vi "串口调试程序.VI"() -> ()   [LabVIEW 2015]
uses:
  <vilib>/Instr/_visa.llb/VISA Configure Serial Port (Instr).vi
panel:
  out "当前时间":timestamp
  in  "清零":bool
  out "接收字节数":u32
  out "发送字节数":u32
  in  "Boolean 9":bool
  in  "毫秒倍数":u32=100 min=2 step=1
  in  "自动发送":bool
  in  "十六进制发送":bool
  in  "OK Button 2":bool
  in  "十六进制接收":bool
  in  "Boolean 8":bool
  in  "退出":bool
  out "接收数据区：":string
  in  "发送数据区：":string
  in  "发送":bool
  in  "打开":bool caption="stop"
  in  "校验位：":u16(ring) items=["  无校验", "  奇校验", "  偶校验"]
  in  "波特率：":u16(ring)=11 items=["   300", "   600", "   1200", "   2400", "   4800   ", "   9600", "   19200", "   38400", "   43000", "   56000", "   57600", "   115200"]
  in  "通讯口：":u16(ring) items=["   com1", "   com2", "   com3", "   com4", "   com5"]
  # "通讯口设置："
  # "接收数据设置："
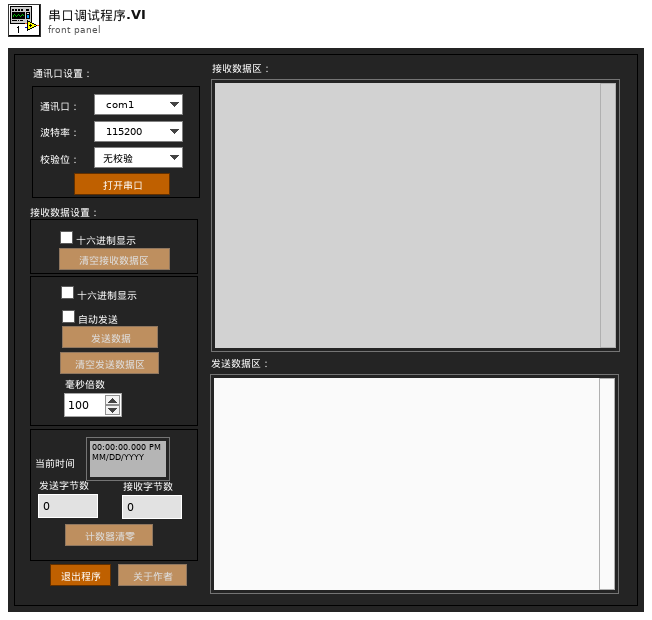
[diagram p1: front panel]
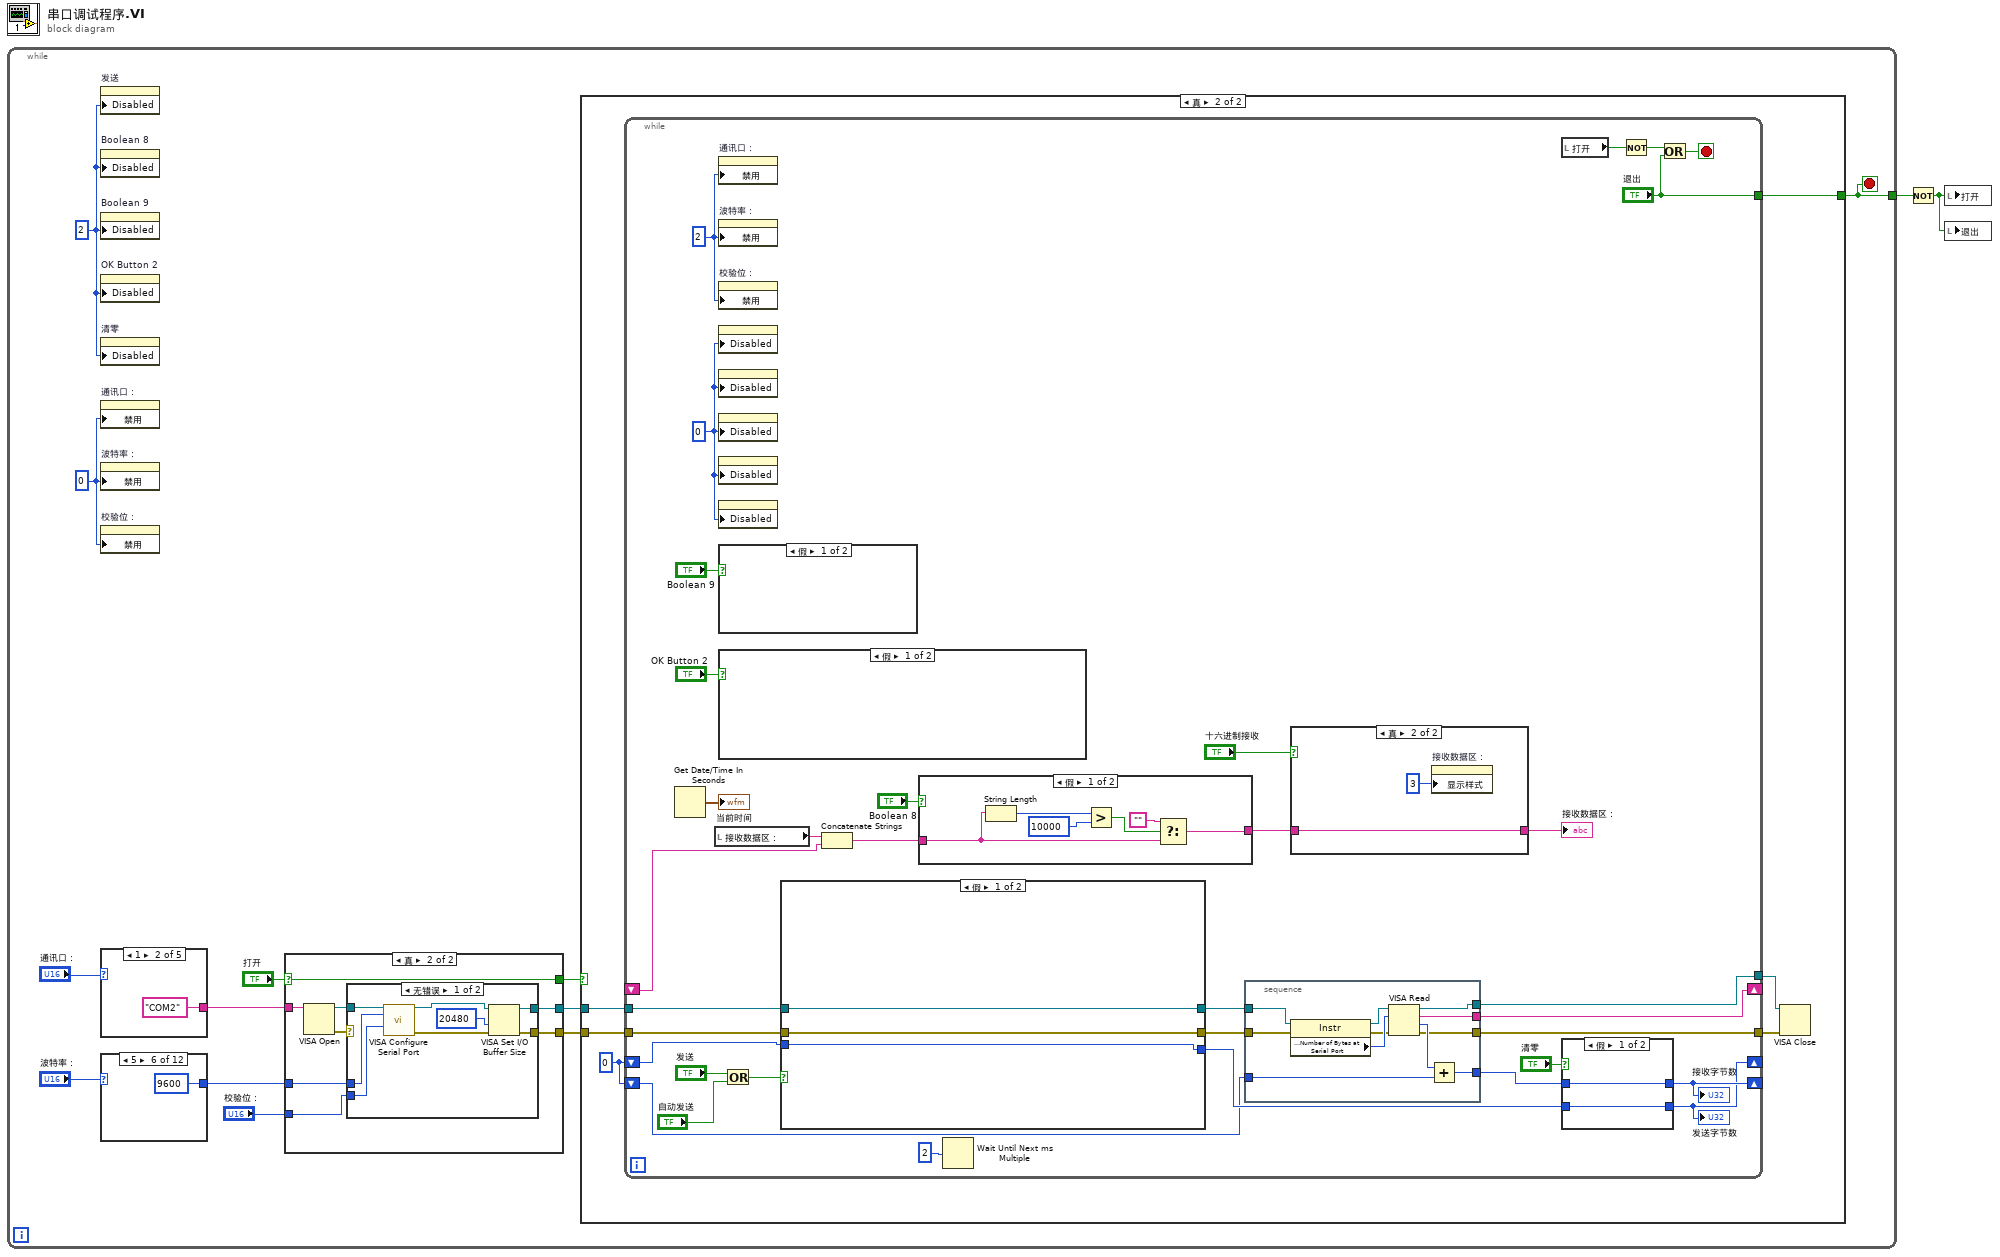
[diagram p0: block diagram]
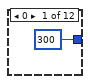
[diagram p2: hidden frame]
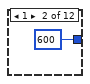
[diagram p3: hidden frame]
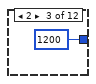
[diagram p4: hidden frame]
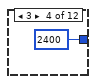
[diagram p5: hidden frame]
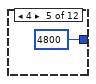
[diagram p6: hidden frame]
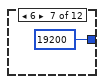
[diagram p7: hidden frame]
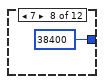
[diagram p8: hidden frame]
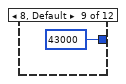
[diagram p9: hidden frame]
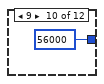
[diagram p10: hidden frame]
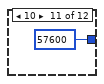
[diagram p11: hidden frame]
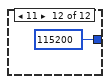
[diagram p12: hidden frame]
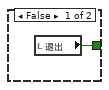
[diagram p13: hidden frame]
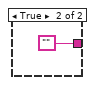
[diagram p14: hidden frame]
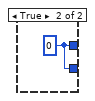
[diagram p15: hidden frame]
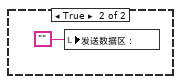
[diagram p16: hidden frame]
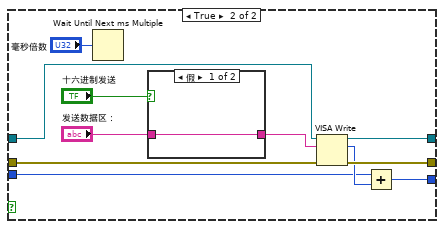
[diagram p17: hidden frame]
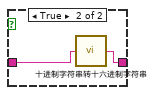
[diagram p18: hidden frame]
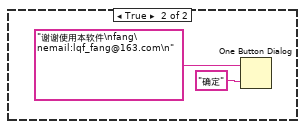
[diagram p19: hidden frame]
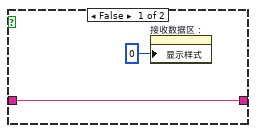
[diagram p20: hidden frame]
diagram:
  n1 = while {
    tunnel: [w7] -> w2
    stop <- w7 stop-if-true
    w5 = 2
    w9 = 0
    n2 = property on="发送" class="Bool"("Disabled"=w5) -> ()  [unwired: 2 in, 2 out]
    n3 = property on="Boolean 8" class="Bool"("Disabled"=w5) -> ()  [unwired: 2 in, 2 out]
    n4 = property on="Boolean 9" class="Bool"("Disabled"=w5) -> ()  [unwired: 2 in, 2 out]
    n5 = property on="OK Button 2" class="Bool"("Disabled"=w5) -> ()  [unwired: 2 in, 2 out]
    n6 = property on="清零" class="Bool"("Disabled"=w5) -> ()  [unwired: 2 in, 2 out]
    n7 = property on="通讯口：" class="Ring (严格)"("禁用"=w9) -> ()  [unwired: 2 in, 2 out]
    n8 = property on="波特率：" class="Ring (严格)"("禁用"=w9) -> ()  [unwired: 2 in, 2 out]
    n9 = property on="校验位：" class="Ring (严格)"("禁用"=w9) -> ()  [unwired: 2 in, 2 out]
    n10 = case shown="1" "通讯口：" {
      tunnel: ["COM1" "COM2" "COM3" "COM4" "COM5"] -> w8
      frame 0, Default {
      }
      frame 1 {
      }
      frame 2 {
      }
      frame 3 {
      }
      frame 4 {
      }
    }
    n11 = case shown="5" "波特率：" {
      tunnel: [300 600 1200 2400 4800 9600 19200 38400 43000 56000 57600 115200] -> w3
      frame 0 {
      }
      frame 1 {
      }
      frame 2 {
      }
      frame 3 {
      }
      frame 4 {
      }
      frame 5 {
      }
      frame 6 {
      }
      frame 7 {
      }
      frame 8, Default {
      }
      frame 9 {
      }
      frame 10 {
      }
      frame 11 {
      }
    }
    n12 = case shown="真" "打开" {
      selector: "打开" -> [w113 w121]
      tunnel: w3 -> [_ w117]
      tunnel: [w113 w121] -> w12
      tunnel: [_ w115] -> w11
      tunnel: [_ w114] -> w10
      tunnel: w8 -> [_ w120]
      tunnel: "校验位：" -> [_ w116]
      frame False {
      }
      frame True {
        n13 = VISA Open(VISA resource name=w120) -> (VISA resource name=w118:refnum<visa-resource-name>, error out=w119:errorcluster)  [unwired: 4 in]
        n14 = case shown="无错误" w119 {
          tunnel: w118 -> [w129 _]
          tunnel: w117 -> [w128 _]
          tunnel: w116 -> [w127 _]
          tunnel: [w123 _] -> w115
          tunnel: [w124 _] -> w114
          frame No Error {
            n15 = call-poly "VISA Configure Serial Port"("VISA resource name"=w129, "baud rate (9600)"=w128, "parity (0:none)"=w127) -> ("VISA resource name out"=w126:refnum<visa-resource-name>, "error out"=w125:errorcluster)  [unwired: 11 in]
            n16 = VISA Set I/O Buffer Size(VISA resource name=w126, size (4096)=u32 20480 ("大小(4096)"), error in (no error)=w125) -> (VISA resource name out=w123:refnum<visa-resource-name>, error out=w124:errorcluster)  [unwired: 1 in]
          }
          frame Error {
            n17 = One Button Dialog(message="ERROR!" ("消息")) -> ()  [unwired: 1 in, 1 out]
          }
        }
      }
    }
    n18 = case shown="真" w12 {
      tunnel: w11 -> [_ w33]
      tunnel: w10 -> [_ w32]
      tunnel: [w27 w29] -> w7
      frame False {
        n19 = local read "退出"() -> (w27:bool)
      }
      frame True {
        w28 = 0
        n20 = while {
          shift-right: [w67] -> _
          shift-left: _ -> [w65]
          tunnel: w33 -> [w61]
          tunnel: w32 -> [w60]
          tunnel: ["退出"] -> w29
          tunnel: [w54] -> w31
          tunnel: [w53] -> w30
          shift-right: [w39] -> _
          shift-left: w28 -> [w37]
          shift-right: [w38] -> _
          shift-left: w28 -> [w40]
          stop <- w51 stop-if-true
          w42 = 0
          w59 = 2
          n21 = Get Date/Time In Seconds() -> (seconds since 1Jan1904=→"当前时间":timestamp)
          n22 = local read "接收数据区："() -> (w66:string)
          n23 = property on="通讯口：" class="Ring (严格)"("禁用"=w59) -> ()  [unwired: 2 in, 2 out]
          n24 = property on="波特率：" class="Ring (严格)"("禁用"=w59) -> ()  [unwired: 2 in, 2 out]
          n25 = property on="校验位：" class="Ring (严格)"("禁用"=w59) -> ()  [unwired: 2 in, 2 out]
          n26 = property on="发送" class="Bool"("Disabled"=w42) -> ()  [unwired: 2 in, 2 out]
          n27 = property on="Boolean 8" class="Bool"("Disabled"=w42) -> ()  [unwired: 2 in, 2 out]
          n28 = property on="Boolean 9" class="Bool"("Disabled"=w42) -> ()  [unwired: 2 in, 2 out]
          n29 = property on="OK Button 2" class="Bool"("Disabled"=w42) -> ()  [unwired: 2 in, 2 out]
          n30 = property on="清零" class="Bool"("Disabled"=w42) -> ()  [unwired: 2 in, 2 out]
          n31 = case shown="假" "Boolean 9" {
            frame False {
            }
            frame True {
              n32 = local write "发送数据区："("") -> ()
            }
          }
          n33 = case shown="假" "OK Button 2" {
            frame False {
            }
            frame True {
              n34 = One Button Dialog(message="谢谢使用本软件\nfang\nemail:lqf_fang@163.com\n", button name ("OK")="确定") -> ()  [unwired: 1 out]
            }
          }
          n35 = Or(x="发送", y="自动发送") -> (x .or. y?=w55:bool)
          n36 = case shown="假" w55 {
            tunnel: w61 -> [w92 w103]
            tunnel: w60 -> [w91 w102]
            tunnel: [w92 w101] -> w58
            tunnel: [w91 w100] -> w57
            tunnel: w40 -> [w90 w94]
            tunnel: [w90 w93] -> w44
            frame False {
            }
            frame True {
              n37 = Wait Until Next ms Multiple(millisecond multiple="毫秒倍数") -> ()  [unwired: 1 out]
              n38 = case shown="假" "十六进制发送" {
                tunnel: "发送数据区：" -> [w104 w106]
                tunnel: [w104 w105] -> w98
                frame False {
                }
                frame True {
                  n39 = call "十进制字符串转十六进制字符串.vi"("字符串"=w106) -> ("电子表格字符串"=w105:string)
                }
              }
              n40 = VISA Write(VISA resource name=w103, write buffer=w98, error in (no error)=w102) -> (VISA resource name out=w101:refnum<visa-resource-name>, return count=w95:u32, error out=w100:errorcluster)
              n41 = Add(x=w94, y=w95) -> (x+y=w93:u32)
            }
          }
          n42 = Concatenate Strings(w66, w65) -> (w35:string)
          n43 = case shown="假" "Boolean 8" {
            tunnel: [w69 ""] -> w34
            tunnel: w35 -> [w70 _]
            frame False {
              n44 = String Length(string=w70) -> (length=w73:i32)
              n45 = Greater?(x=w73, y=10000) -> (0:w71:bool)
              n46 = Select(t="", s=w71, f=w70) -> (s? t:f=w69:string)
            }
            frame True {
            }
          }
          n47 = Wait Until Next ms Multiple(millisecond multiple=u32 2 ("毫秒倍数")) -> ()  [unwired: 1 out]
          n48 = stacked-sequence {
            tunnel: w58 -> [w89]
            tunnel: w57 -> [w86]
            tunnel: [w84] -> w67
            tunnel: [w83] -> w54
            tunnel: [w80] -> w53
            tunnel: [w81] -> w43
            tunnel: w37 -> [w79]
            frame #0 {
              n49 = property class="Instr"(reference=w89, error in=w86) -> (reference out=w87:refnum<visa-resource-name>, error out=w85:errorcluster, "Serial Settings:Number of Bytes at Serial Port"=w88:u32)
              n50 = VISA Read(VISA resource name=w87, byte count=w88, error in (no error)=w85) -> (VISA resource name out=w83:refnum<visa-resource-name>, read buffer=w84:string, return count=w82:u32, error out=w80:errorcluster)
              n51 = Add(x=w82, y=w79) -> (x+y=w81:u32)
            }
          }
          n52 = case shown="真" "十六进制接收" {
            tunnel: [w109 w111] -> w63
            tunnel: w34 -> [w109 w111]
            frame False {
              n53 = property on="接收数据区：" class="Str"("显示样式"=0) -> ()  [unwired: 2 in, 2 out]
            }
            frame True {
              n54 = property on="接收数据区：" class="Str"("显示样式"=3) -> ()  [unwired: 2 in, 2 out]
            }
          }
          "接收数据区：" <- w63
          n55 = local read "打开"() -> (w49:bool)
          n56 = case shown="假" "清零" {
            tunnel: [w76 w77] -> w38
            tunnel: w44 -> [w76 _]
            tunnel: w43 -> [w75 _]
            tunnel: [w75 w77] -> w39
            frame False {
            }
            frame True {
              w77 = 0
            }
          }
          "发送字节数" <- w38
          "接收字节数" <- w39
          n57 = Not(x=w49) -> (.not. x?=w48:bool)
          n58 = Or(x=w48, y="退出") -> (x .or. y?=w51:bool)
        }
        n59 = VISA Close(VISA resource name=w31, error in (no error)=w30) -> ()  [unwired: 1 out]
      }
    }
  }
  n60 = Not(x=w2) -> (.not. x?=w1:bool)
  n61 = local write "打开"(w1) -> ()
  n62 = local write "退出"(w1) -> ()
